vi "Feeder Pickup.vi"(8 "error in (no error)":errorcluster) -> ()   [LabVIEW 2014]
uses:
  Main/Robot Global Data.vi
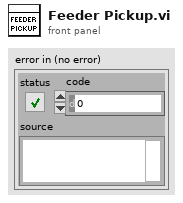
[diagram p1: front panel]
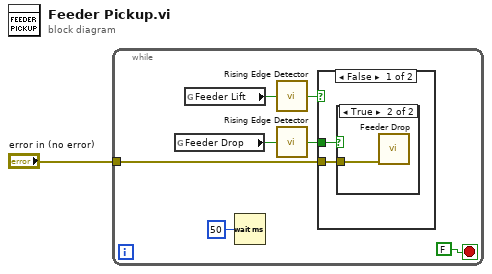
[diagram p0: block diagram]
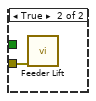
[diagram p3: hidden frame]
diagram:
  n1 = while {
    tunnel: "error in (no error)" -> [w3]
    stop <- FALSE stop-if-true
    n2 = global read "Robot Global Data.vi" "Feeder Drop"() -> (w7:bool)
    n3 = global read "Robot Global Data.vi" "Feeder Lift"() -> (w6:bool)
    n4 = Wait (ms)(milliseconds to wait=u32 50) -> ()  [unwired: 1 out]
    n5 = call "Rising Edge Detector.vi"("Input"=w6) -> ("Rising edge?"=w5:bool)
    n6 = call "Rising Edge Detector.vi"("Input"=w7) -> ("Rising edge?"=w4:bool)
    n7 = case shown="False" w5 {
      tunnel: w4 -> [w10 _]
      tunnel: w3 -> [w9 w12]
      frame False {
        n8 = case shown="True" w10 {
          tunnel: w9 -> [_ w11]
          frame False {
          }
          frame True {
            n9 = call "Feeder Drop.vi"("error in (no error)"=w11) -> ()  [unwired: 10 in, 1 out]
          }
        }
      }
      frame True {
        n10 = call "Feeder Lift.vi"("error in (no error)"=w12) -> ()  [unwired: 10 in, 1 out]
      }
    }
  }
